vi "Create.vi"(7 "Direction":T1, 8 "error in (no error)":errorcluster, 9 "Custom Config Data":u8[](array[numeric]), 10 "Name":string, 11 "CIF_Fifo_Raw_Multi in":refnum<class "CIF_NIChn_Raw.lvclass">) -> (0 "error out":errorcluster, 3 "CIF_Fifo_Raw_Multi out":refnum<class "CIF_NIChn_Raw.lvclass">)   [LabVIEW 2021, in "CIF_NIChn_Raw.lvclass"]
doc: "This will create a U8 channel of the channel type provided by the type override. This is needed to support linking of different classes of FIFOs or to provide a new class that only creates a new type."
uses:
  CIF_NIChn_Raw.lvclass
  D:/dev/Packages/Channel_Manager/src/CIFChannels/CIFChannels.lvclass
  D:/dev/Packages/Channel_Manager/src/CIF_NIChn/NIChn/CIF_NIChn.lvclass
  D:/dev/Packages/Channel_Manager/src/CIF_NIChn/FIFO_U8/CIF_NIChn_Fifo_U8.lvclass
  CIFChannels/Typedef/Direction.ctl
  CIFChannels/Typedef/Disconnect Behavior.ctl
  CIFChannels/CIFChannels.lvclass/CIFChannels.ctl
  CIF_NIChn_Raw.lvclass/CIF_NIChn_Raw.ctl
  <vilib>/CIF Foundation/CIF Utilities/Statistics/I64/Stats_I64_CIF_U.lvclass/Stats_I64_CIF_U.ctl
  CIFChannels/Typedef/Channel State.ctl
  NIChn/CIF_NIChn.lvclass/CIF_NIChn.ctl
  FIFO_U8/CIF_NIChn_Fifo_U8.lvclass/CIF_NIChn_Fifo_U8.ctl
  1ff93ec1-b9a6-44e7-8b99-fa7cc07c6703.vi
  CIFChannels/Accessors/Write Channel State.vi
  NIChn/Accessors/Write CIF Channel.vi
  CIFChannels/Accessors/Write Channel Benchmark.vi
  CIFChannels/Accessors/Write Flatten Benchmark.vi
  FIFO_U8/Accessors/Write Payload.vi
  CIFChannels/Accessors/Write Type.vi
  CIFChannels/SubVIs/Get Type from Class.vi
  ChannelCommon/Utilities/Unflatten FIFO Config.vi
  CIFChannels/Utilities/Apply Flags.vi
  CIFChannels/Accessors/Write Channel Class.vi
  CIFChannels/Accessors/Write Direction.vi
  CIFChannels/Accessors/Write Tag Disconnect Behavior.vi
  CIFChannels/Accessors/Write Name.vi
  CIFChannels/Accessors/Write Custom Config Data.vi
  <vilib>/CIF Foundation/NI Channels/SubVIs/Add Error.vi
  1ff93ec1-b9a6-44e7-8b99-fa7cc07c6703.vi/c28b0ead-42ad-4072-80a2-aca7f2bd7ce3.vi
  <vilib>/CIF Foundation/NI Channels/SubVIs/CIFServices Fill In Error Info Ex.vi
  <vilib>/CIF Foundation/NI Channels/SubVIs/Get dll Path.vi
  <vilib>/CIF Foundation/CIF Utilities/DataTypes/Unflatten U64.vi
  ChannelCommon/Utilities/Expand FIFO Flags.vi
  <vilib>/CIF Foundation/CIF Utilities/Errors/Append Error Location.vi
  <vilib>/Utility/LVClass/Get LV Class Name.vi
  <vilib>/CIF Foundation/CIF Utilities/Statistics/I64/Stats_I64_CIF_U.lvclass
  CIFChannels/CIFChannels.lvclass
  ChannelCommon/ChannelCommon.lvlib
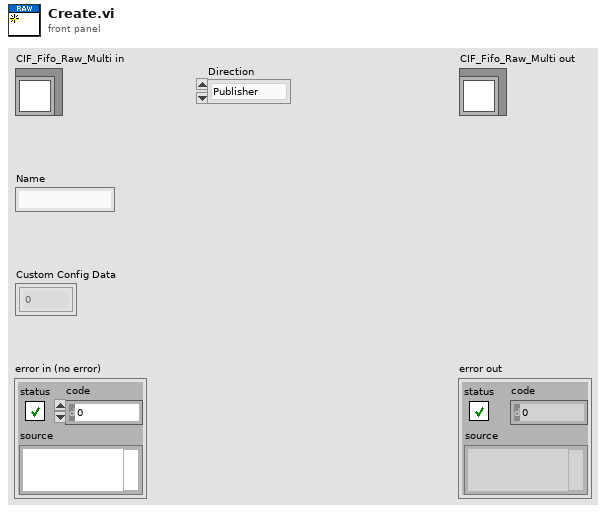
[diagram p1: front panel]
types:
  T1 = typedef "CIFChannels.lvclass/Direction.ctl" = enum16{"Publisher", "Subscriber"}
  T2 = typedef "CIFChannels.lvclass/Disconnect Behavior.ctl" = enum16{"Default value", "Last value", "Error with default"}
  T3 = typedef "CIFChannels.lvclass/Channel State.ctl" = enum16{"Creating", "Disconnected", "Connecting", "Connected", "Destroyed"}
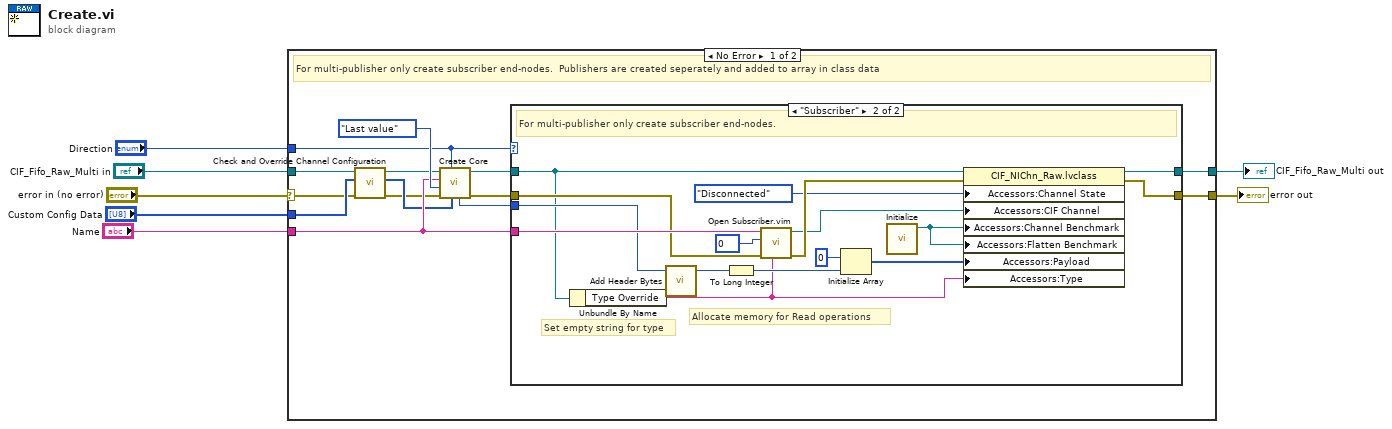
[diagram p0: block diagram]
diagram:
  n1 = case shown="No Error" "error in (no error)" {
    selector: "error in (no error)" -> [w15 w41]
    tunnel: [w9 w41] -> w3
    tunnel: [w10 w40] -> w1
    tunnel: "CIF_Fifo_Raw_Multi in" -> [w18 w40]
    tunnel: "Name" -> [w20 _]
    tunnel: "Direction" -> [w12 _]
    tunnel: "Custom Config Data" -> [w17 _]
    frame No Error {
      # "For multi-publisher only create subscriber end-nodes.  Publishers are created seperately and added to array in class data"
      n2 = call-dynamic "Check and Override Channel Configuration.vi"("error in (no error)"=w15, "Custom Config Data in"=w17, "CIFFIFO in"=w18) -> ("error out"=w14:errorcluster, "Custom Config Data out"=w16:u8[], "CIFFIFO out"=w13:refnum<class "CIF_NIChn_Raw.lvclass">)  [unwired: 6 in]
      n3 = call "Create Core.vi"("Custom Config Data"=w16, "Direction"=w12, "error in (no error)"=w14, "Disconnect Behavior"=Disconnect_Behavior."Last value", "Name"=w20, "CIFChannels in"=w13) -> ("error out"=w19:errorcluster, "CIFChannels out"=w11:refnum<class "CIF_NIChn_Raw.lvclass">, "Bytes/Msg"=w8:u64)  [unwired: 1 in, 2 out]
      n4 = case shown="\"Subscriber\"" w12 {
        tunnel: w20 -> [_ w39]
        tunnel: w19 -> [w23 w38]
        tunnel: w11 -> [w22 w25]
        tunnel: [w22 w29] -> w10
        tunnel: [w23 w28] -> w9
        tunnel: w8 -> [_ w27]
        frame "Publisher", Default {
          # "Publishers are created seperately and added to array in class data"
        }
        frame "Subscriber" {
          # "Set empty string for type"
          # "Allocate memory for Read operations"
          # "For multi-publisher only create subscriber end-nodes."
          n5 = Unbundle By Name(w25) -> ("Type Override"=w24:string)
          n6 = call "Add Header Bytes.vi"("Bytes/Msg"=w27) -> ("Bytes/Msg with header"=w26:u64)  [unwired: 3 in]
          n7 = To Long Integer(number=w26) -> (32bit integer=w37:i32)
          n8 = call "Open Subscriber.vim"("Channel Type Description"=w24, "error in"=w38, "Input Type"=u8 0, "Channel Name"=w39) -> ("error out"=w33:errorcluster, "CIF Channel"=w31:refnum<k21>)  [unwired: 6 in]
          n9 = Initialize Array(u8 0 ("Numeric"), w37) -> (w30:u8[])
          n10 = call <vilib>:"Initialize.vi"() -> ("Stats_I64_CIF_U out"=w34:refnum<class "Stats_I64_CIF_U.lvclass">)  [unwired: 10 in, 1 out]
          n11 = property class="CIF_NIChn_Raw.lvclass"(reference=w25, error in=w33, "Accessors:Channel State"=Channel_State."Disconnected" ("Channel State"), "Accessors:CIF Channel"=w31, "Accessors:Channel Benchmark"=w34, "Accessors:Flatten Benchmark"=w34, "Accessors:Payload"=w30, "Accessors:Type"=w24) -> (reference out=w29:refnum<class "CIF_NIChn_Raw.lvclass">, error out=w28:errorcluster)
        }
      }
    }
    frame Error {
    }
  }
  "error out" <- w3
  "CIF_Fifo_Raw_Multi out" <- w1
